vi "Get Size of Data from TD - Path - Returns Correct Size.vi"() -> ()   [LabVIEW 2017, in "Composition.Tests.lvlib"]
uses:
  Composition.Tests.lvlib
  <vilib>/addons/_JKI Toolkits/Caraya/classes/Assert/Assert Equal Value_Variant.vi
  Composition/Composition.lvlib
  <vilib>/addons/_JKI Toolkits/Caraya/classes/Assert/Assert.lvclass
  <vilib>/addons/_JKI Toolkits/Caraya/classes/Test/Test.lvclass
panel:
  out "error out":errorcluster
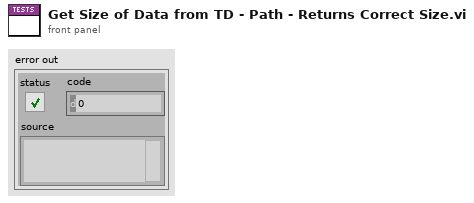
[diagram p1: front panel]
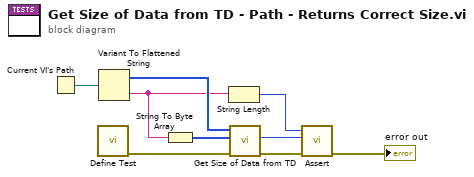
[diagram p0: block diagram]
diagram:
  n1 = Current VI's Path() -> (path=w1:path)
  n2 = call <vilib>:"Define Test.vi"() -> ("error out"=w2:errorcluster)  [unwired: 11 in]
  n3 = Variant To Flattened String(Variant=w1) -> (data string=w6:string, 1:w9:i16[])
  n4 = String To Byte Array(string=w6) -> (unsigned byte array=w8:u8[])
  n5 = String Length(string=w6) -> (length=w3:i32)
  n6 = call "Get Size of Data from TD.vi"("error in (no error)"=w2, "Data String"=w8, "Type Descriptor"=w9) -> ("error out"=w7:errorcluster, "Size of Data"=w4:i32)  [unwired: 7 in]
  n7 = call-poly <vilib>:"Assert.vi"("error in (no error)"=w7, "Y"=w4, "X"=w3) -> ("error out"=→"error out":errorcluster)  [unwired: 8 in]
